vi "4275A_Auto_Range_On.vi"(8 "error in":errorcluster) -> (0 "error out":errorcluster)   [LabVIEW 2020]
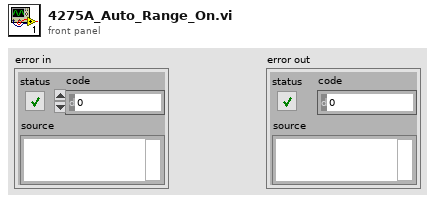
[diagram p1: front panel]
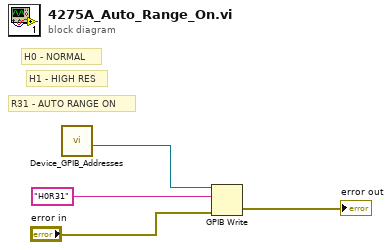
[diagram p0: block diagram]
diagram:
  # "H1 - HIGH RES"
  # "H0 - NORMAL"
  # "R31 - AUTO RANGE ON"
  n1 = call "Device_GPIB_Addresses.vi"() -> ("HP 4275A Address"=w1:refnum<visa-resource-name>)  [unwired: 9 in, 2 out]
  n2 = GPIB Write(0:w1, 1:"H0R31" ("address string"), 3:"error in") -> (6:→"error out":errorcluster)  [unwired: 2 in, 1 out]
